vi "Release Notifiers and Queues.vi"(8 "error in (no error)":errorcluster, 11 "Task Base in":refnum<class "Task Base.lvclass">) -> (0 "error out":errorcluster, 3 "Task Base out":refnum<class "Task Base.lvclass">)   [LabVIEW 2023, in "HAL GOOP4.lvlib" / "Task Base.lvclass"]
doc: "Don't call this VI until Do.vi is stopped and all Data Queues and Data Notifiers are read and terminated."
uses:
  Task Base.lvclass
  Task Base.lvclass/Task Base.ctl
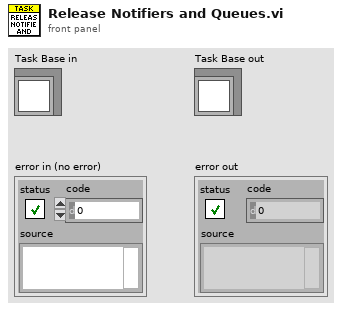
[diagram p1: front panel]
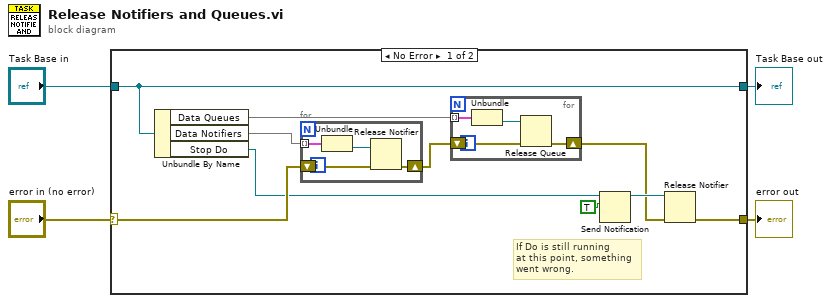
[diagram p0: block diagram]
diagram:
  n1 = case shown="No Error" "error in (no error)" {
    selector: "error in (no error)" -> [w13 w24]
    tunnel: [w9 w24] -> w3
    tunnel: [w14 w23] -> w1
    tunnel: "Task Base in" -> [w14 w23]
    frame No Error {
      # "If Do is still running\nat this point, something\nwent wrong."
      n2 = Unbundle By Name(w14) -> ("Data Queues"=w11:map{string, refnum<queue>}, "Data Notifiers"=w12:map{string, refnum<notifier>}, "Stop Do"=w8:refnum<notifier>)
      n3 = for {
        tunnel: w12 -> [w21] mode=indexing
        shift-right: [w19] -> w10
        shift-left: w13 -> [w22]
        n4 = Unbundle(w21) -> ("Data"=w20:refnum<notifier>)  [unwired: 1 out]
        n5 = Release Notifier(notifier=w20, error in (no error)=w22) -> (error out=w19:errorcluster)  [unwired: 1 in, 2 out]
      }
      n6 = for {
        tunnel: w11 -> [w17] mode=indexing
        shift-right: [w16] -> w5
        shift-left: w10 -> [w18]
        n7 = Unbundle(w17) -> ("Data Queue"=w15:refnum<queue>)  [unwired: 1 out]
        n8 = Release Queue(queue=w15, error in (no error)=w18) -> (error out=w16:errorcluster)  [unwired: 1 in, 2 out]
      }
      n9 = Send Notification(notification=TRUE, notifier=w8) -> (notifier out=w7:refnum<notifier>)  [unwired: 1 in, 1 out]
      n10 = Release Notifier(notifier=w7, error in (no error)=w5) -> (error out=w9:errorcluster)  [unwired: 1 in, 2 out]
    }
    frame Error {
    }
  }
  "error out" <- w3
  "Task Base out" <- w1
